vi "test.vi"() -> ()   [LabVIEW 2022 SP3]
panel:
  out "error out":errorcluster
  in  "error in":errorcluster
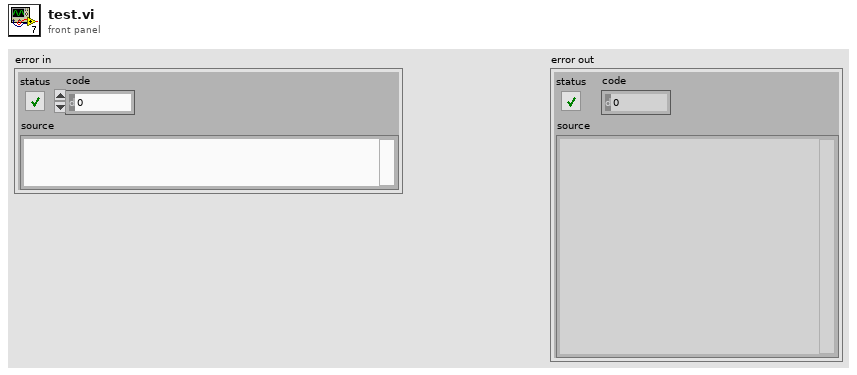
[diagram p1: front panel]
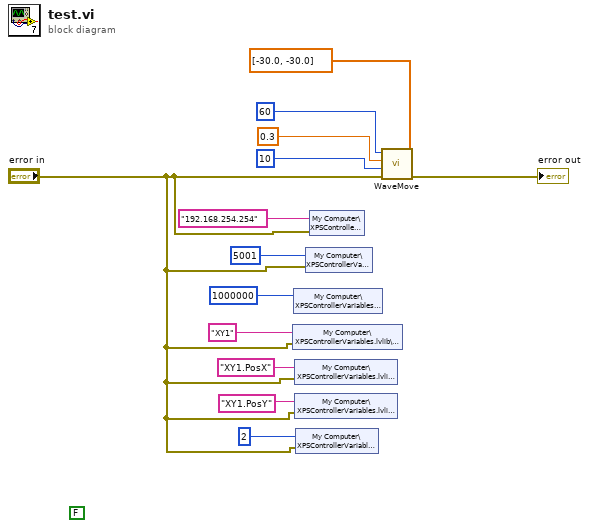
[diagram p0: block diagram]
diagram:
  (unwired) FALSE
  n1 = shared-variable "My Computer\\XPSControllerVariables.lvlib\\GroupName"("XY1", error in="error in") -> ()  [unwired: 1 out]
  n2 = shared-variable "My Computer\\XPSControllerVariables.lvlib\\Timeout"(1000000) -> ()  [unwired: 1 in, 1 out]
  n3 = shared-variable "My Computer\\XPSControllerVariables.lvlib\\PosNameX"("XY1.PosX", error in="error in") -> ()  [unwired: 1 out]
  n4 = shared-variable "My Computer\\XPSControllerVariables.lvlib\\PosNameY"("XY1.PosY", error in="error in") -> ()  [unwired: 1 out]
  n5 = shared-variable "My Computer\\XPSControllerVariables.lvlib\\nbitem"(2, error in="error in") -> ()  [unwired: 1 out]
  n6 = shared-variable "My Computer\\XPSControllerVariables.lvlib\\Port"(5001, error in="error in") -> ()  [unwired: 1 out]
  n7 = shared-variable "My Computer\\XPSControllerVariables.lvlib\\IP"("192.168.254.254", error in="error in") -> ()  [unwired: 1 out]
  n8 = call "WaveMove.vi"("Length"=60, "Spacing"=0.3, "LineNo"=10, "error in"="error in", "StartPos"=dbl[] [-30.0, -30.0]) -> ("error out"=→"error out":errorcluster)  [unwired: 5 in]
